vi "init.vi"(8 "error in (no error)":errorcluster, 11 "ForceSensor in":refnum<class "ForceSensorCalculator.lvclass">) -> (0 "error out":errorcluster, 3 "ForceSensor out":refnum<class "ForceSensorCalculator.lvclass">)   [LabVIEW 2013, in "ForceSensorCalculator.lvlib" / "ForceSensorCalculator.lvclass"]
uses:
  <userlib>/Common/Devices/ForceSensorCalculator/ForceSensorCalculator/ForceSensorCalculator.lvclass
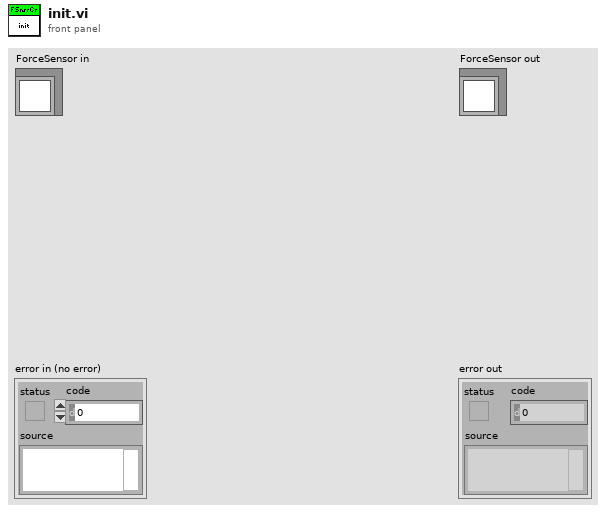
[diagram p1: front panel]
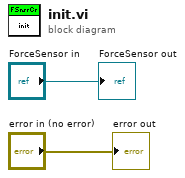
[diagram p0: block diagram]
diagram:
  "error out" <- "error in (no error)"
  "ForceSensor out" <- "ForceSensor in"
